vi "gety.vi"() -> ()   [LabVIEW 2014]
uses:
  <resource>/Framework/Providers/LVClassLibrary/NewAccessors/MemberVICreation.lvlib
panel:
  in  "Path":path=path "E:/Projects/8205/Trunk/LVCM.lvproj"
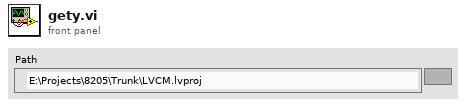
[diagram p1: front panel]
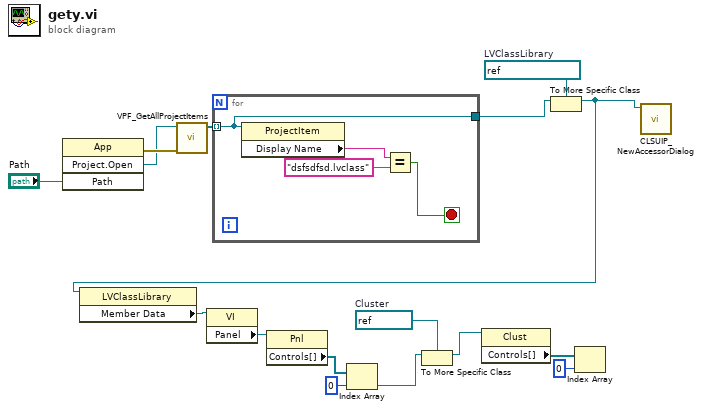
[diagram p0: block diagram]
diagram:
  w5 = refnum<vi> refnum  # Cluster
  w11 = refnum<vi> refnum  # LVClassLibrary
  n1 = invoke class="App" method="Project.Open"("Path"="Path") -> (error out=w16:errorcluster, "Project:Open"=w15:refnum<vi>)  [unwired: 3 in, 2 out]
  n2 = call <resource>:"VPF_GetAllProjectItems.vi"("error in (no error)"=w16, "ProjectRefNum"=w15) -> ("All Project Items"=w14:refnum<vi>[])  [unwired: 5 in, 4 out]
  n3 = for {
    tunnel: w14 -> [w17] mode=indexing
    tunnel: [w17] -> w12
    stop <- w18 stop-if-true
    n4 = property class="ProjectItem"(reference=w17) -> ("Display Name"=w20:string)  [unwired: 1 in, 2 out]
    n5 = Equal?(x=w20, y="dsfsdfsd.lvclass") -> (x = y?=w18:bool)
  }
  n6 = To More Specific Class(target class=w11, reference=w12) -> (specific class reference=w1:refnum<vi>)  [unwired: 1 in, 1 out]
  n7 = property class="LVClassLibrary"(reference=w1) -> ("Member Data"=w10:refnum<vi>)  [unwired: 1 in, 2 out]
  n8 = property class="VI"(reference=w10) -> ("Panel"=w9:refnum<vi>)  [unwired: 1 in, 2 out]
  n9 = property class="Pnl"(reference=w9) -> ("Controls[]"=w8:refnum<vi>[])  [unwired: 1 in, 2 out]
  n10 = Index Array(array=w8, index=0) -> (element=w4:refnum<vi>)
  n11 = To More Specific Class(target class=w5, reference=w4) -> (specific class reference=w6:refnum<vi>)  [unwired: 1 in, 1 out]
  n12 = property class="Clust"(reference=w6) -> ("Controls[]"=w3:refnum<vi>[])  [unwired: 1 in, 2 out]
  n13 = Index Array(array=w3, index=0) -> ()  [unwired: 1 out]
  n14 = call <resource>:"CLSUIP_NewAccessorDialog.vi"("DNL_LVClassLibrary Refnum"=w1) -> ()  [unwired: 8 in, 3 out]
